vi "Add PV Value.vi"(7 "PV name":string, 8 "error in":errorcluster, 10 "Value in":refnum<class "Value.lvclass">, 11 "Server in":refnum<class "Server.lvclass">) -> (0 "error out":errorcluster, 3 "Server out":refnum<class "Server.lvclass">)   [LabVIEW 2020, in "Server.lvlib" / "Server.lvclass"]
uses:
  Server.lvclass
  Value/Value/Value.lvclass
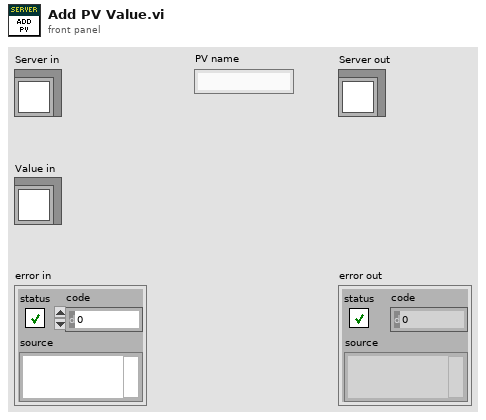
[diagram p1: front panel]
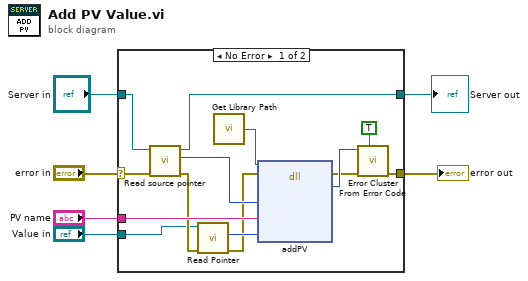
[diagram p0: block diagram]
diagram:
  n1 = case shown="No Error" "error in" {
    selector: "error in" -> [w20 w22]
    tunnel: [w11 w22] -> w4
    tunnel: [w16 w21] -> w5
    tunnel: "Server in" -> [w19 w21]
    tunnel: "PV name" -> [w15 _]
    tunnel: "Value in" -> [w7 _]
    frame No Error {
      n2 = call "Read source pointer.vi"("error in (no error)"=w20, "Server in"=w19) -> ("error out"=w8:errorcluster, "source pointer"=w17:i64, "Server out"=w16:refnum<class "Server.lvclass">)  [unwired: 7 in]
      n3 = call-dynamic "Read Pointer.vi"("error in (no error)"=w8, "Value in"=w7) -> ("error out"=w9:errorcluster, "pointer"=w10:i64)  [unwired: 7 in, 1 out]
      n4 = call "Get Library Path.vi"() -> ("Path"=w18:path)  [unwired: 1 in]
      n5 = dll-call lib="?" fn="addPV"(path in=w18, error in=w9, "source"=w17, "pv_name"=w15, "value"=w10) -> (error out=w12:errorcluster, "ret_code"=w13:i32)  [unwired: 4 in, 1 out]
      n6 = call <vilib>:"Error Cluster From Error Code.vi"("show call chain? (False)"=TRUE, "error in (no error)"=w12, "error code (0)"=w13) -> ("error out"=w11:errorcluster)  [unwired: 6 in]
    }
    frame Error {
    }
  }
  "error out" <- w4
  "Server out" <- w5
